vi "StrToArray.vi"(8 "error in":errorcluster caption="错误输入", 11 "StrIn":string) -> (0 "error out":errorcluster caption="错误输出", 3 "ArrayOut":string[](array[string]))   [LabVIEW 2013]
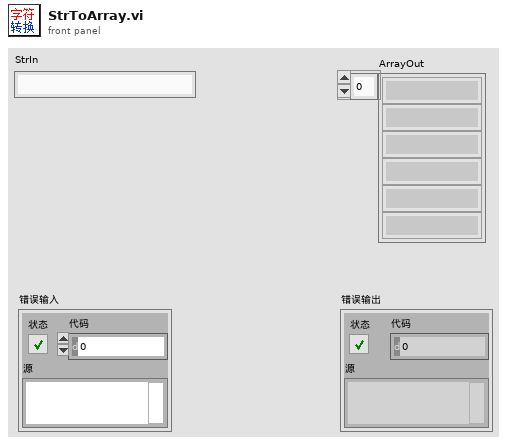
[diagram p1: front panel]
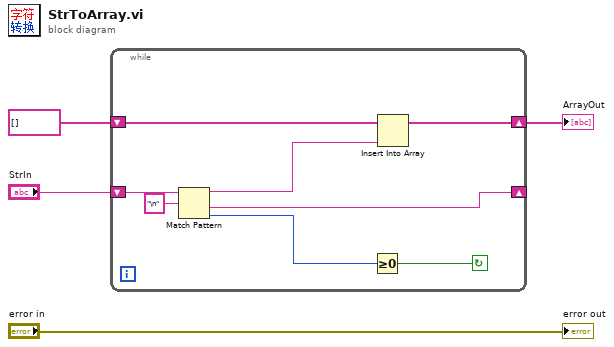
[diagram p0: block diagram]
diagram:
  n1 = while {
    shift-right: [w6] -> w2
    shift-left: string[] [] -> [w8]
    shift-right: [w11] -> _
    shift-left: "StrIn" -> [w12]
    stop <- w9 continue-if-true
    n2 = Match Pattern(string=w12, regular expression="\n") -> (before substring=w7:string, after substring=w11:string, offset past match=w10:i32)  [unwired: 1 in, 1 out]
    n3 = Greater Or Equal To 0?(x=w10) -> (x >= 0?=w9:bool)
    n4 = Insert Into Array(array=w8, new element=w7) -> (w6:string[])  [unwired: 1 in]
  }
  "ArrayOut" <- w2
  "error out" <- "error in"
